vi "BIO_set_fd.vi"(8 "error in (no error)":errorcluster, 9 "Close on free? (T)":bool=TRUE, 10 "socket fd":i32, 11 "BIO in":refnum<class "BIO.lvclass">) -> (0 "error out":errorcluster, 3 "BIO out":refnum<class "BIO.lvclass">)   [LabVIEW 2013, in "OpenSSL Socket.lvlib" / "BIO.lvclass"]
uses:
  BIO.lvclass
  SSL-Lib/SSL-Lib.lvclass/SSL-Lib.ctl
  BIO.lvclass/BIO.ctl
  SSL-Lib/Read Crypto Library Path.vi
  Read Handle.vi
  SSL-Lib/SSL-Lib.lvclass
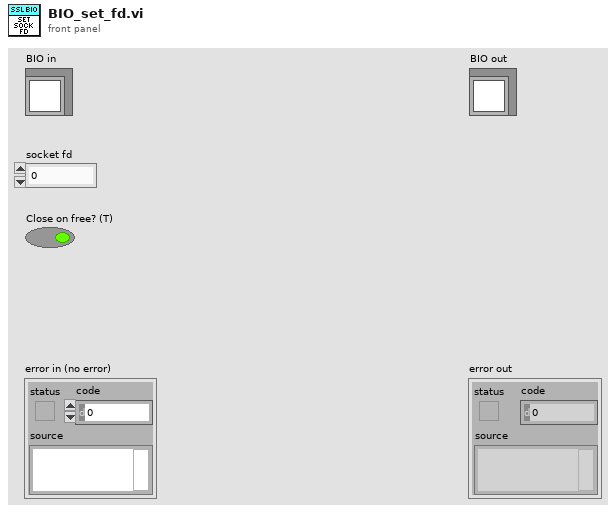
[diagram p1: front panel]
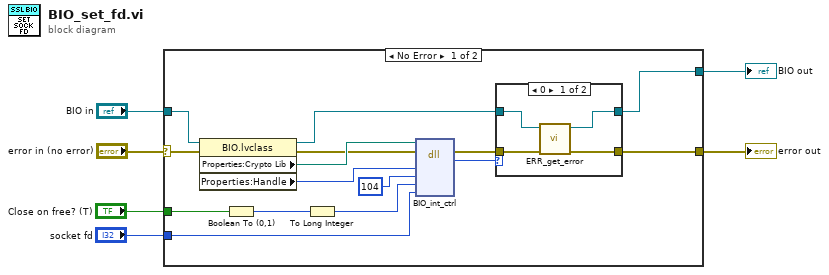
[diagram p0: block diagram]
diagram:
  n1 = case shown="No Error" "error in (no error)" {
    selector: "error in (no error)" -> [w19 w29]
    tunnel: [w11 w29] -> w5
    tunnel: [w12 w28] -> w3
    tunnel: "BIO in" -> [w20 w28]
    tunnel: "socket fd" -> [w10 _]
    tunnel: "Close on free? (T)" -> [w7 _]
    frame No Error {
      n2 = property class="BIO.lvclass"(reference=w20, error in=w19) -> (reference out=w13:refnum<class "BIO.lvclass">, error out=w16:errorcluster, "Properties:Crypto Lib"=w18:path, "Properties:Handle"=w17:u64)
      n3 = Boolean To (0,1)(Boolean=w7) -> (0, 1=w9:i16)
      n4 = To Long Integer(number=w9) -> (32bit integer=w8:i32)
      n5 = dll-call lib="C:/Program Files (x86)/National Instruments/Shared/nissl/NIlibeay32.dll" fn="BIO_int_ctrl"(path in=w18, error in=w16, "BIO"=w17, "cmd"=104, "larg"=w8, "parg"=w10) -> (error out=w14:errorcluster, "return type"=w15:i32)  [unwired: 5 in, 1 out]
      n6 = case shown="0" w15 {
        tunnel: w14 -> [w25 w27]
        tunnel: [w22 w27] -> w11
        tunnel: w13 -> [w24 w26]
        tunnel: [w23 w26] -> w12
        frame 0 {
          n7 = call "ERR_get_error.vi"("error in (no error)"=w25, "SSL-Lib in"=w24) -> ("error out"=w22:errorcluster, "SSL-Lib out"=w23:refnum<class "BIO.lvclass">)  [unwired: 8 in]
        }
        frame Default {
        }
      }
    }
    frame Error {
    }
  }
  "error out" <- w5
  "BIO out" <- w3
